vi "Gear Down.vi"(3 "Step":i32, 4 "Acceptable Error":dbl, 5 "Startup":bool) -> (0 "Completed":bool, 1 "Output":dbl)   [LabVIEW 2016]
uses:
  Command Execution State.ctl
  Rotation/Rotation Globals.vi
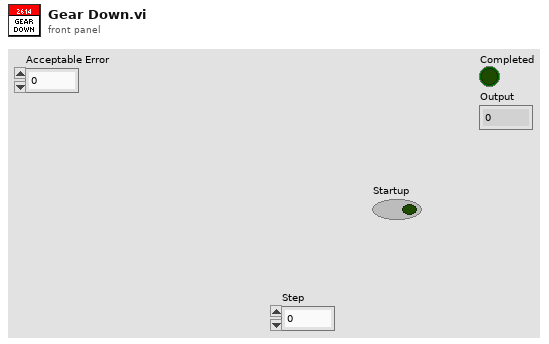
[diagram p1: front panel]
types:
  T1 = typedef "Command Execution State.ctl" = enum16{"Initialize", "Execute", "Finish"}
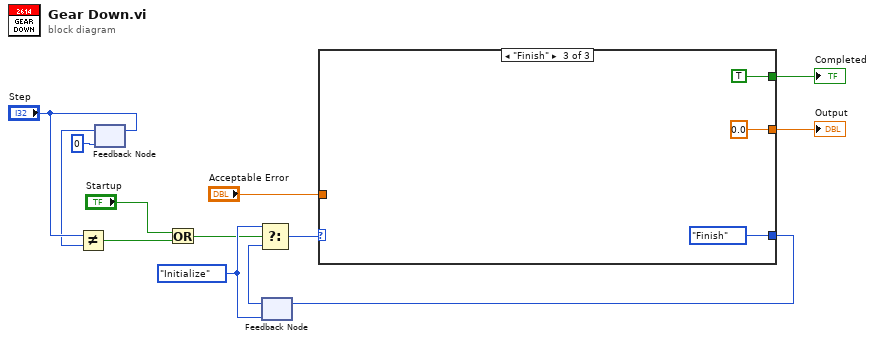
[diagram p0: block diagram]
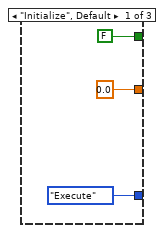
[diagram p2: hidden frame]
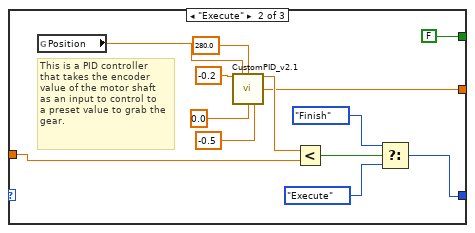
[diagram p3: hidden frame]
diagram:
  w9 = Command_Execution_State."Initialize" ("Play State")
  n1 = feedback #1(0 ("Step")) -> (w4:i32)
  n2 = Not Equal?(x="Step", y=w4) -> (x != y?=w2:bool)
  n3 = feedback-in #1("Step") -> ()
  n4 = Or(x="Startup", y=w2) -> (x .or. y?=w3:bool)
  n5 = feedback #2(w9) -> (w10:T1)
  n6 = Select(t=w9, s=w3, f=w10) -> (s? t:f=w13:T1)
  n7 = case shown="\"Finish\"" w13 {
    tunnel: [Command_Execution_State."Execute" ("Play State") w29 Command_Execution_State."Finish" ("Play State")] -> w11
    tunnel: [FALSE FALSE TRUE] -> w8
    tunnel: "Acceptable Error" -> [_ w19 _]
    tunnel: [0.0 ("Command") w17 0.0 ("Command")] -> w6
    frame "Initialize", Default {
    }
    frame "Execute" {
      # "This is a PID controller\nthat takes the encoder\nvalue of the motor shaft\nas an input to control to\na preset value to grab the\ngear."
      n8 = global read "Rotation Globals.vi" "Position"() -> (w24:dbl)
      n9 = call "CustomPID_v2.1.vi"("Kp"=-0.2, "Process Variable"=w24, "Goal"=280.0, "Max Ouput"=0.0, "Min Output"=-0.5) -> ("Current Error"=w20:dbl, "Command"=w17:dbl)  [unwired: 8 in, 1 out]
      n10 = Less?(x=w20, y=w19) -> (x < y?=w18:bool)
      n11 = Select(t=Command_Execution_State."Finish" ("Play State"), s=w18, f=Command_Execution_State."Execute" ("Play State")) -> (s? t:f=w29:T1)
    }
    frame "Finish" {
    }
  }
  "Completed" <- w8
  "Output" <- w6
  n12 = feedback-in #2(w11) -> ()
